vi "Set MLJ Stage Home.vi"(8 "error in (no error)":errorcluster, 10 "Cluster in":T1, 11 "MLJ Reference In":refnum<k24>) -> (0 "error out":errorcluster, 2 "Cluster out":T1, 3 "MLJ Reference Out":refnum<k24>)   [LabVIEW 2017]
uses:
  Controls/Translation Stage Cluster.ctl
  General/Controls/Translation Stage Types.ctl
  C:/Users/OCT/Documents/SSOCT/SerialSectOCT/Software/Thorlabs.MotionControl.Controls.dll
  Thorlabs.MotionControl.Controls.dll
  C:/Users/OCT/Documents/SSOCT/SerialSectOCT/Software/Thorlabs.MotionControl.IntegratedStepperMotorsCLI.dll
  Thorlabs.MotionControl.IntegratedStepperMotorsCLI.dll
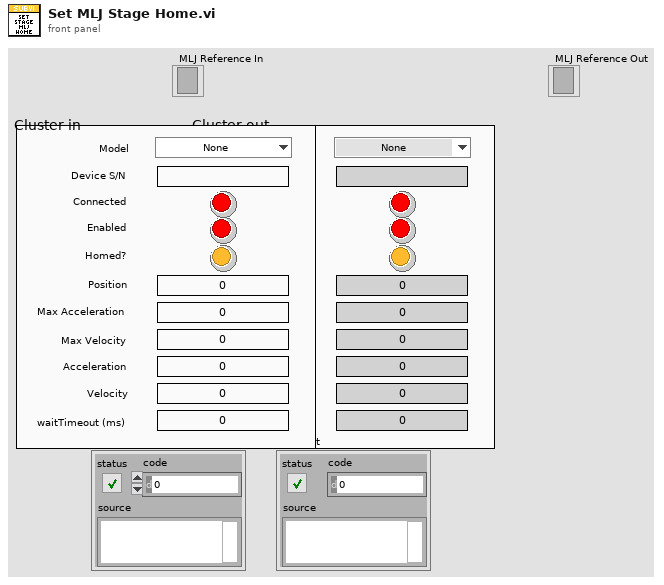
[diagram p1: front panel]
types:
  T1 = typedef "Translation Stage Cluster.ctl" = cluster{"Position":dbl, "Is.Enabled?":bool, "Is.Connected?":bool, "Device SN":string, "AccelerationMaximum":dbl, "VelocityMaximum":dbl, "Acceleration":dbl, "Velocity":dbl, "waitTimeout (ms)":i32, "Model":T2, "Is.Homed?":bool}
  T2 = typedef "Translation Stage Types.ctl" = enum16{"None", "Thorlabs LTS", "Thorlabs MLJ"}
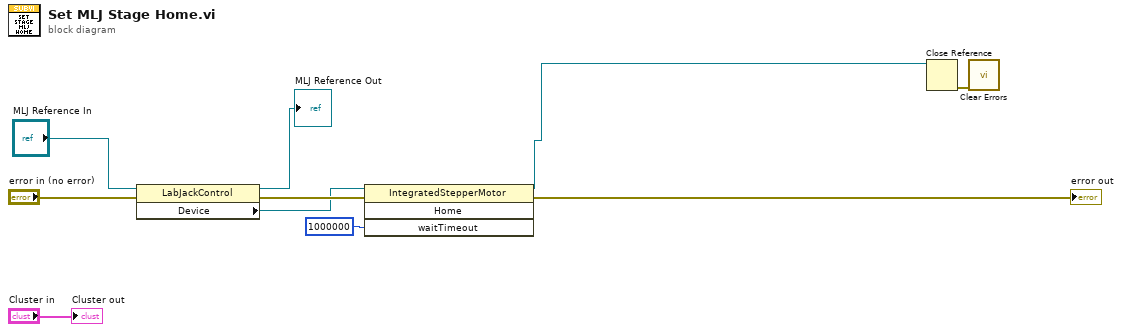
[diagram p0: block diagram]
diagram:
  n1 = property class="LabJackControl"(reference="MLJ Reference In", error in="error in (no error)") -> (reference out=→"MLJ Reference Out":refnum<k24>, error out=w5:errorcluster, "Device"=w4:refnum<k24>)
  n2 = invoke class="IntegratedStepperMotor" method="Home"(reference=w4, error in=w5, "waitTimeout"=1000000) -> (reference out=w1:refnum<k24>, error out=→"error out":errorcluster)  [unwired: 1 in, 2 out]
  n3 = Close Reference(reference=w1) -> (error out=w3:errorcluster)  [unwired: 1 in]
  n4 = call <vilib>:"Clear Errors.vi"("error in (no error)"=w3) -> ()  [unwired: 5 in, 2 out]
  "Cluster out" <- "Cluster in"
